vi "Launcher Top Level.vi"   [LabVIEW 2015]
uses:
  Controller/Controller/Controller.lvclass
  <vilib>/ActorFramework/Actor/Actor.lvclass
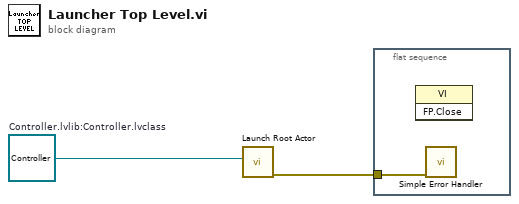
[diagram p0: block diagram]
diagram:
  w2 = refnum<class "Controller.lvclass"> refnum  # Controller.lvlib:Controller.lvclass
  n1 = call <vilib>:"Launch Root Actor.vi"("Actor"=w2) -> ("error out"=w1:errorcluster)  [unwired: 9 in, 1 out]
  n2 = flat-sequence {
    tunnel: w1 -> [w3]
    frame #0 {
      n3 = invoke class="VI" method="FP.Close"() -> ()  [unwired: 3 in, 3 out]
      n4 = call <vilib>:"Simple Error Handler.vi"("error in (no error)"=w3) -> ()  [unwired: 4 in, 5 out]
    }
  }
